vi "Identity Value.vi"(3 "Log Manager Identity in":refnum<class "Log Manager Identity.lvclass">) -> (1 "Value":string)   [LabVIEW 2020, in "VolatusData.lvlib" / "Log Manager Identity.lvclass"]
uses:
  Log Manager Identity.lvclass
  Log Manager Identity.lvclass/Log Manager Identity.ctl
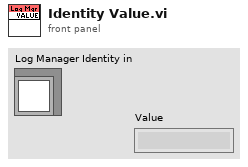
[diagram p1: front panel]
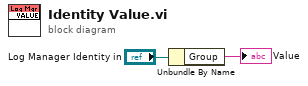
[diagram p0: block diagram]
diagram:
  n1 = Unbundle By Name("Log Manager Identity in") -> ("Group"=→"Value":string)
